vi "graph_data.vi"(1 "datetime_to":string="2026-07-07", 2 "datetime_from":string="2026-07-01", 3 "sensor ID":u32=3917) -> (0 "value":T1)   [LabVIEW 2024]
uses:
  API_Key.vi
  <vilib>/httpClient/LabVIEWHTTPClient.lvlib
panel:
  out "Is_wrong_Key":bool
  out "headers":string
  out "body":string
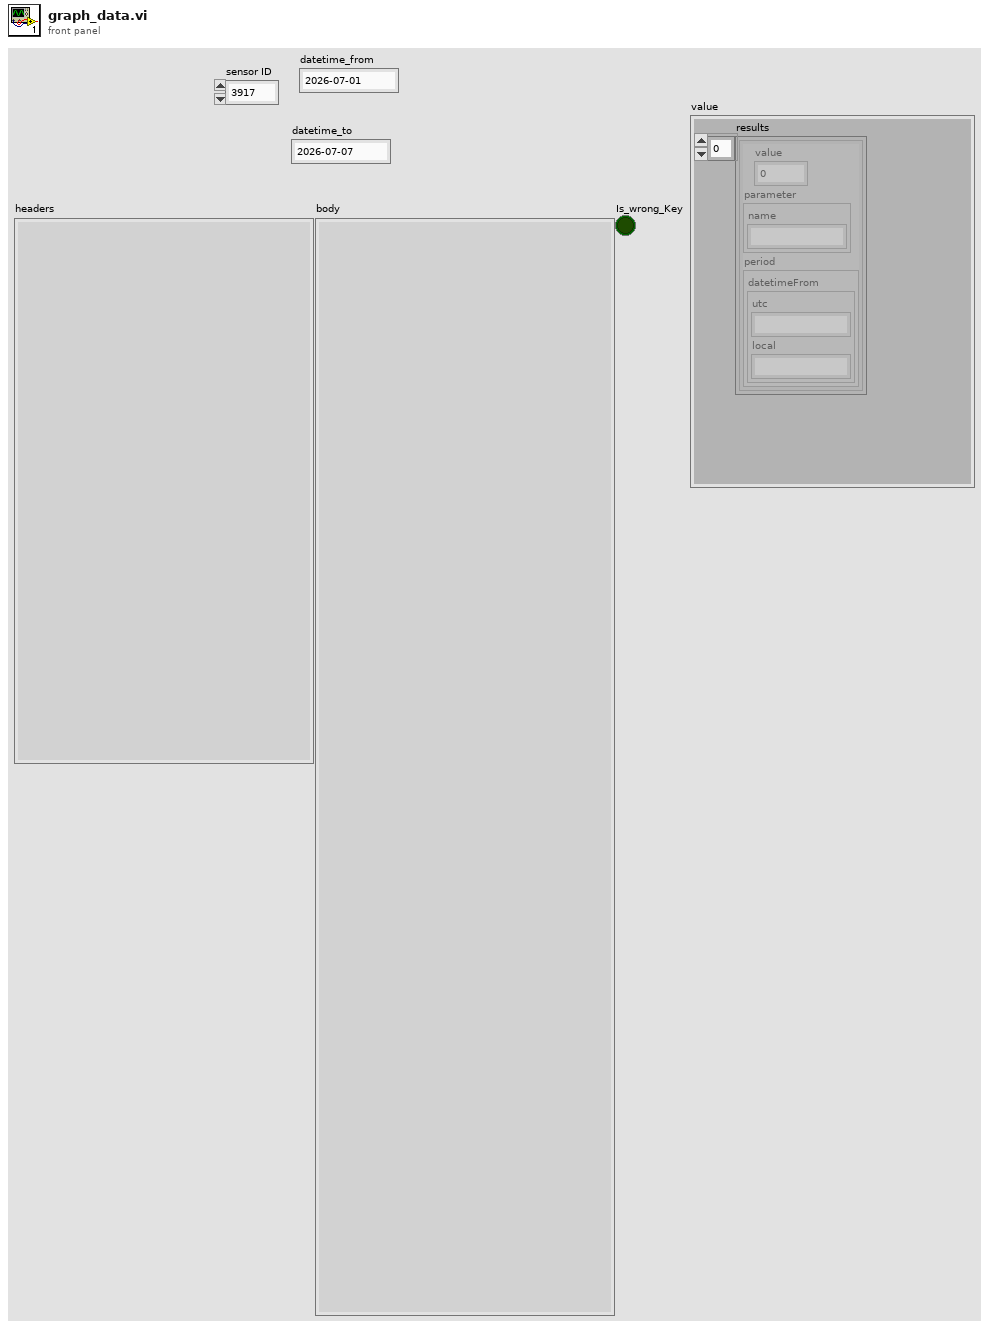
[diagram p1: front panel]
types:
  T1 = cluster{"results":cluster{"value":dbl, "parameter":cluster{"name":string}, "period":cluster{"datetimeFrom":cluster{"utc":string, "local":string}}}[]}
  T2 = typedef "LabVIEWHTTPClient.lvlib/ClientHandle.ctl" = refnum<k1>
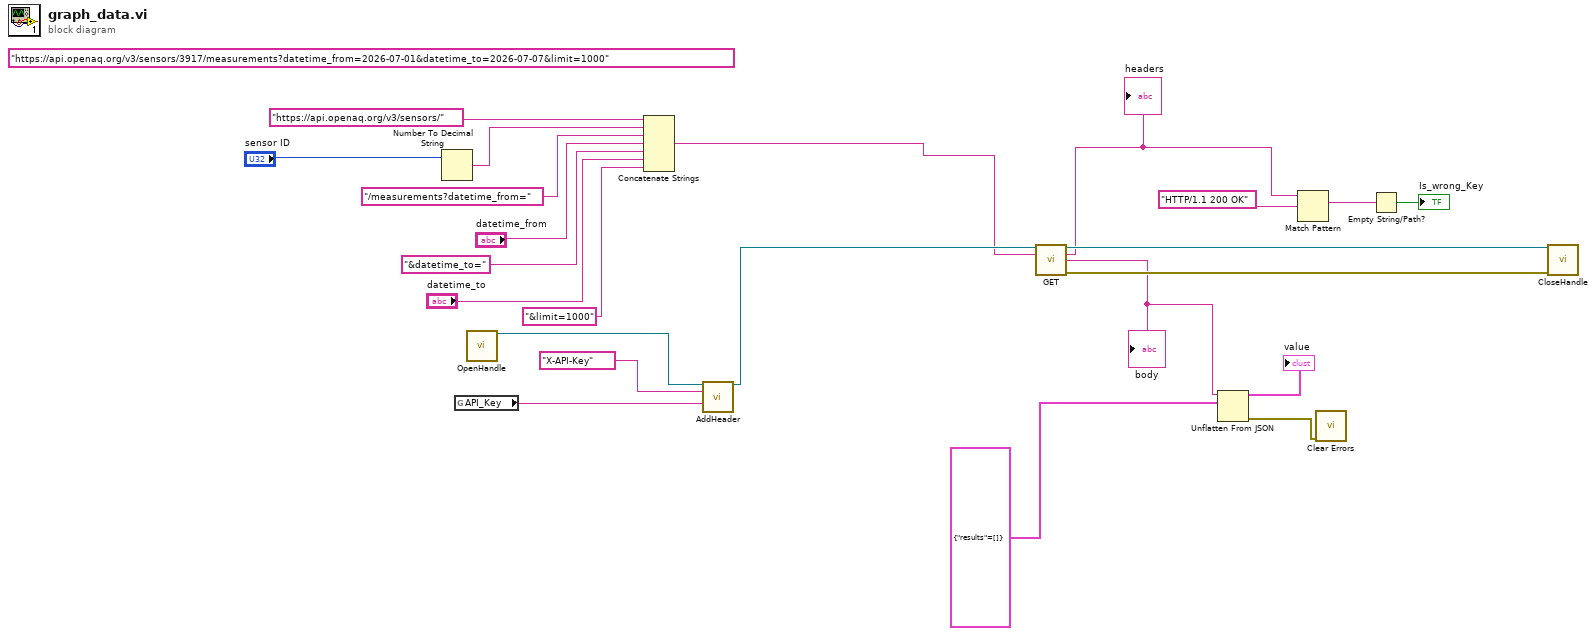
[diagram p0: block diagram]
diagram:
  (unwired) "https://api.openaq.org/v3/sensors/3917/measurements?datetime_from=2026-07-01&datetime_to=2026-07-07&limit=1000"
  n1 = Number To Decimal String(number="sensor ID") -> (decimal integer string=w8:string)  [unwired: 1 in]
  n2 = global read "API_Key.vi" "API_Key"() -> (w1:string)
  n3 = call <vilib>:"OpenHandle.vi"() -> ("client handle out"=w21:T2)  [unwired: 14 in, 1 out]
  n4 = Concatenate Strings("https://api.openaq.org/v3/sensors/" ("string"), w8, "/measurements?datetime_from=", "datetime_from", "&datetime_to=", "datetime_to", "&limit=1000") -> (w2:string)
  n5 = call <vilib>:"AddHeader.vi"("client handle"=w21, "header"="X-API-Key", "value"=w1) -> ("client handle out"=w19:T2)  [unwired: 11 in, 1 out]
  n6 = call <vilib>:"GET.vi"("client handle"=w19, "url"=w2) -> ("client handle out"=w23:T2, "headers"=w18:string, "body"=w14:string, "error out"=w22:errorcluster)  [unwired: 10 in]
  "body" <- w14
  "headers" <- w18
  n7 = Unflatten From JSON(JSON string=w14, type and defaults=T1 {"results"=[]}) -> (value=→"value":T1, error out=w12:errorcluster)  [unwired: 5 in]
  n8 = Match Pattern(string=w18, regular expression="HTTP/1.1 200 OK") -> (match substring=w16:string)  [unwired: 1 in, 3 out]
  n9 = call <vilib>:"Clear Errors.vi"("error in (no error)"=w12) -> ()  [unwired: 5 in, 2 out]
  n10 = Empty String/Path?(string/path=w16) -> (empty?=→"Is_wrong_Key":bool)
  n11 = call <vilib>:"CloseHandle.vi"("client handle"=w23, "error in (no error)"=w22) -> ()  [unwired: 13 in, 1 out]
